vi "RT Loop - DAQ Control.vi"(11 "Message Queue":refnum<queue> caption="消息队列") -> ()   [LabVIEW 2013]
doc: "该DAQ控制循环VI对4路输入通道并行地进行控制计算，将结果输出至输出通道。"
uses:
  support/Message Queue/Message Cluster.ctl
  <vilib>/Platform/TimedLoop/XDataNode/timing_clust.ctl
  <vilib>/Platform/TimedLoop/XDataNode/nitl_modes.ctl
  <vilib>/Platform/TimedLoop/XDataNode/wakeup.ctl
  controls/Functional Global Operation.ctl
  controls/Control State.ctl
  Globals/Global - Configuration Options.vi
  <vilib>/Platform/TimedLoop/XDataNode/XDataNode.xnode
  <vilib>/Platform/TimedLoop/XDataNode/XDNodeRunTimeDep.lvlib
  support/Message Queue/Message Queue.lvlib
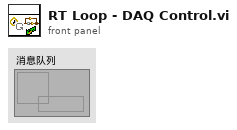
[diagram p1: front panel]
types:
  T1 = typedef "DAQ Tasks.ctl" = cluster{"AI Task":refnum<k21>, "AO Task":refnum<k21>}
  T2 = typedef "Functional Global Operation.ctl" = enum16{"Initialize", "Read", "Write"}
  T3 = typedef "XDNodeRunTimeDep.lvlib/timing_clust.ctl" = cluster{"Expected End [f-1]":u64, "Actual End [f-1]":u64, "Finished Late? [f-1]":bool, "Expected End [i-1]":u64, "Actual End [i-1]":u64, "Finished Late? [i-1]":bool, "Expected Start [i]":u64, "Actual Start [i]":u64, "Expected Start [f]":u64, "Actual Start [f]":u64, "Source Name":string, "Structure Name":string, "Period":i64, "Deadline":i64, "Offset":i64, "Start":i64, "Priority":i32, "Timeout":i32, "Mode":T4, "Wakeup Reason":T5, "Error":errorcluster, "Source Type":string, "Secondary Source Type":string, "Global End Time":u64, "Global Start Time":u64, "Frame Duration":u64, "Iteration Duration":u64, "Assigned CPU":i32, "I/O Scan Engine Mode":u32}
  T4 = typedef "XDNodeRunTimeDep.lvlib/nitl_modes.ctl" = enum32{"No Change", "Process missed periods, maintain original phase", "Discard missed periods, maintain original phase", "Process missed periods, ignore original phase", "Discard missed periods, ignore original phase"}
  T5 = typedef "XDNodeRunTimeDep.lvlib/wakeup.ctl" = enum32{"Normal", "Aborted", "Asynchronous wakeup", "Timing source error", "Timed loop error", "Timeout"}
  T6 = typedef "Control State.ctl" = enum16{"Safe State", "Manual", "Control (PID)"}
  T7 = typedef "Control Configuration.ctl" = cluster{"PID Gains":cluster{"proportional gain (Kc)":dbl, "integral gain (Kc*Ts/Ti)":dbl, "derivative gain (Kc*Td/Ts)":dbl}, "Output Range":cluster{"output high":dbl, "output low":dbl}}
  T8 = cluster{"proportional gain (Kc)":dbl, "integral gain (Kc*Ts/Ti)":dbl, "derivative gain (Kc*Td/Ts)":dbl}
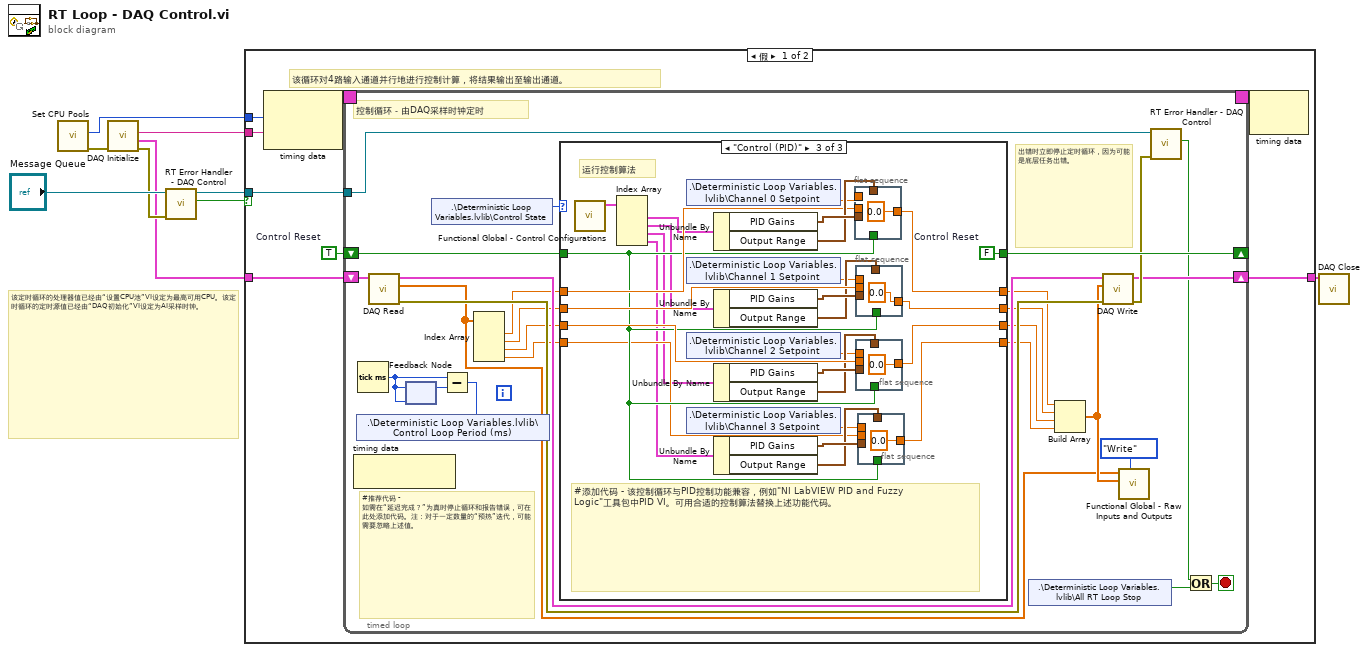
[diagram p0: block diagram]
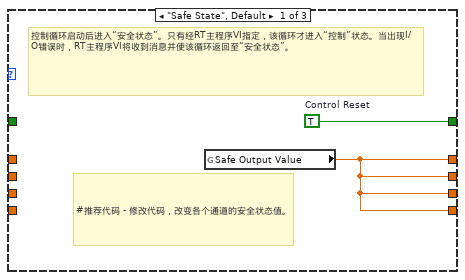
[diagram p2: hidden frame]
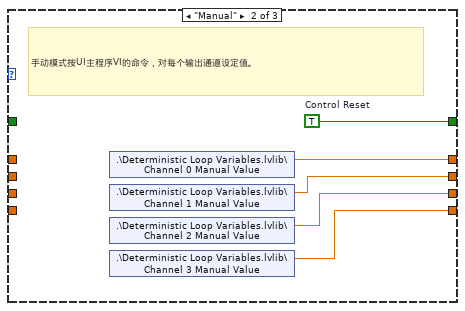
[diagram p3: hidden frame]
diagram:
  # "该定时循环的处理器值已经由“设置CPU池”VI设定为最高可用CPU。该定时循环的定时源值已经由“DAQ初始化”VI设定为AI采样时钟。"
  n1 = call "Set CPU Pools.vi"() -> ("error out"=w3:errorcluster, "Processor Assignment"=w2:i32)  [unwired: 10 in]
  n2 = call "DAQ Initialize.vi"("error in (no error)"=w3) -> ("error out"=w7:errorcluster, "DAQ Tasks"=w5:T1, "Timing Source"=w6:string)  [unwired: 8 in]
  n3 = call "RT Error Handler - DAQ Control.vi"("error in (no error)"=w7, "Message Queue"="Message Queue") -> ("Enqueued Error?"=w1:bool, "dup Message Queue"=w8:refnum<queue>)  [unwired: 8 in]
  n4 = case shown="假" w1 {
    tunnel: w8 -> [w14 _]
    tunnel: w6 -> [w13 _]
    tunnel: w5 -> [w12 w89]
    tunnel: [w11 w89] -> w4
    tunnel: w2 -> [w10 _]
    frame False {
      w15 = TRUE  # Control Reset
      # "该循环对4路输入通道并行地进行控制计算，将结果输出至输出通道。"
      n5 = node-c288(w10, w13) -> (w17:T3)
      n6 = timed-loop {
        shift-right: [w43] -> _
        shift-left: w15 -> [w42]
        timing: w17 -> [_]
        timing-out: [_] -> w16
        tunnel: w14 -> [w41]
        shift-right: [w31] -> w11
        shift-left: w12 -> [w33]
        stop <- w19 stop-if-true
        # "出错时立即停止定时循环，因为可能是底层任务出错。"
        # "#推荐代码 - 如需在“延迟完成？”为真时停止循环和报告错误，可在此处添加代码。注：对于一定数量的“预热”迭代，可能需要忽略上述值。"
        # "控制循环－由DAQ采样时钟定时"
        n7 = node-c288() -> ()  [unwired: 1 in, 1 out]
        n8 = Tick Count (ms)() -> (millisecond timer value=w40:u32)
        n9 = call "DAQ Read.vi"("DAQ Tasks"=w33) -> ("error out"=w34:errorcluster, "data"=w20:dbl[], "dup DAQ Tasks"=w32:T1)  [unwired: 8 in]
        n10 = feedback-in #1(w40) -> ()
        n11 = feedback #1(w40) -> (w39:u32)
        n12 = shared-variable ".\\Deterministic Loop Variables.lvlib\\Control State"() -> (w36:T6)  [unwired: 1 in, 1 out]
        n13 = Subtract(x=w40, y=w39) -> (x-y=w37:u32)
        n14 = shared-variable ".\\Deterministic Loop Variables.lvlib\\Control Loop Period (ms)"(w37) -> ()  [unwired: 1 in, 1 out]
        n15 = Index Array(array=w20) -> (element #1=w24:dbl, element #2=w23:dbl, element #3=w22:dbl, element #4=w21:dbl)  [unwired: 4 in]
        n16 = case shown="\"Control (PID)\"" w36 {
          tunnel: w24 -> [_ _ w74]
          tunnel: [w45 w50 w77] -> w28
          tunnel: [w46 w51 w78] -> w43
          tunnel: w42 -> [_ _ w62]
          tunnel: w23 -> [_ _ w73]
          tunnel: w22 -> [_ _ w69]
          tunnel: w21 -> [_ _ w61]
          tunnel: [w45 w49 w71] -> w27
          tunnel: [w45 w48 w66] -> w26
          tunnel: [w45 w47 w63] -> w25
          frame "Safe State", Default {
            w46 = TRUE  # Control Reset
            # "控制循环启动后进入“安全状态”。只有经RT主程序VI指定，该循环才进入“控制”状态。当出现I/O错误时，RT主程序VI将收到消息并使该循环返回至“安全状态”。"
            # "安全状态－下一个状态改变前，输出常量值"
            # "#推荐代码 - 修改代码，改变各个通道的安全状态值。"
            n17 = global read "Global - Configuration Options.vi" "Safe Output Value"() -> (w45:dbl)
          }
          frame "Manual" {
            w51 = TRUE  # Control Reset
            # "手动模式按UI主程序VI的命令，对每个输出通道设定值。"
            # "安全状态－下一个状态改变前，输出常量值"
            n18 = shared-variable ".\\Deterministic Loop Variables.lvlib\\Channel 0 Manual Value"() -> (w50:dbl)  [unwired: 1 in, 1 out]
            n19 = shared-variable ".\\Deterministic Loop Variables.lvlib\\Channel 1 Manual Value"() -> (w49:dbl)  [unwired: 1 in, 1 out]
            n20 = shared-variable ".\\Deterministic Loop Variables.lvlib\\Channel 2 Manual Value"() -> (w48:dbl)  [unwired: 1 in, 1 out]
            n21 = shared-variable ".\\Deterministic Loop Variables.lvlib\\Channel 3 Manual Value"() -> (w47:dbl)  [unwired: 1 in, 1 out]
          }
          frame "Control (PID)" {
            w78 = FALSE  # Control Reset
            # "运行控制算法"
            # "#添加代码 - 该控制循环与PID控制功能兼容，例如\"NI LabVIEW PID and Fuzzy Logic\"工具包中PID VI。可用合适的控制算法替换上述功能代码。"
            n22 = call "Functional Global - Control Configurations.vi"() -> ("Control Configurations out"=w60:T7[])  [unwired: 11 in]
            n23 = Index Array(array=w60) -> (element #1=w59:T7, element #2=w58:T7, element #3=w57:T7, element #4=w56:T7)  [unwired: 4 in]
            n24 = shared-variable ".\\Deterministic Loop Variables.lvlib\\Channel 0 Setpoint"() -> (w52:dbl)  [unwired: 1 in, 1 out]
            n25 = shared-variable ".\\Deterministic Loop Variables.lvlib\\Channel 1 Setpoint"() -> (w53:dbl)  [unwired: 1 in, 1 out]
            n26 = shared-variable ".\\Deterministic Loop Variables.lvlib\\Channel 2 Setpoint"() -> (w54:dbl)  [unwired: 1 in, 1 out]
            n27 = shared-variable ".\\Deterministic Loop Variables.lvlib\\Channel 3 Setpoint"() -> (w55:dbl)  [unwired: 1 in, 1 out]
            n28 = Unbundle By Name(w59) -> ("PID Gains"=w76:T8, "Output Range"=w75:cluster{"output high":dbl, "output low":dbl})
            n29 = Unbundle By Name(w58) -> ("PID Gains"=w72:T8, "Output Range"=w70:cluster{"output high":dbl, "output low":dbl})
            n30 = Unbundle By Name(w57) -> ("PID Gains"=w68:T8, "Output Range"=w67:cluster{"output high":dbl, "output low":dbl})
            n31 = Unbundle By Name(w56) -> ("PID Gains"=w65:T8, "Output Range"=w64:cluster{"output high":dbl, "output low":dbl})
            n32 = flat-sequence {
              tunnel: [0.0 ("output")] -> w77
              tunnel: w76 -> [_]
              tunnel: w75 -> [_]
              tunnel: w74 -> [_]
              tunnel: w62 -> [_]
              tunnel: w52 -> [_]
              frame #0 {
              }
            }
            n33 = flat-sequence {
              tunnel: w73 -> [_]
              tunnel: w72 -> [_]
              tunnel: [0.0 ("output")] -> w71
              tunnel: w70 -> [_]
              tunnel: w62 -> [_]
              tunnel: w53 -> [_]
              frame #0 {
              }
            }
            n34 = flat-sequence {
              tunnel: w69 -> [_]
              tunnel: w68 -> [_]
              tunnel: w67 -> [_]
              tunnel: [0.0 ("output")] -> w66
              tunnel: w62 -> [_]
              tunnel: w54 -> [_]
              frame #0 {
              }
            }
            n35 = flat-sequence {
              tunnel: w65 -> [_]
              tunnel: w64 -> [_]
              tunnel: [0.0 ("output")] -> w63
              tunnel: w62 -> [_]
              tunnel: w61 -> [_]
              tunnel: w55 -> [_]
              frame #0 {
              }
            }
          }
        }
        n36 = shared-variable ".\\Deterministic Loop Variables.lvlib\\All RT Loop Stop"() -> (w38:bool)  [unwired: 1 in, 1 out]
        n37 = Build Array(w28, w27, w26, w25) -> (w29:dbl[])
        n38 = call "DAQ Write.vi"("error in (no error)"=w34, "Outputs"=w29, "DAQ Tasks"=w32) -> ("error out"=w35:errorcluster, "dup DAQ Tasks"=w31:T1)  [unwired: 7 in]
        n39 = call "Functional Global - Raw Inputs and Outputs.vi"("Functional Global Operation (Read)"=Functional_Global_Operation."Write", "Outputs in"=w29, "Inputs in"=w20) -> ()  [unwired: 7 in, 2 out]
        n40 = call "RT Error Handler - DAQ Control.vi"("error in (no error)"=w35, "Message Queue"=w41) -> ("Enqueued Error?"=w18:bool)  [unwired: 8 in, 1 out]
        n41 = Or(x=w18, y=w38) -> (x .or. y?=w19:bool)
      }
      n42 = node-c288(w16) -> ()  [unwired: 1 out]
    }
    frame True {
      # "如设置DAQ任务时出错，不执行定时循环，直接关闭各任务。"
    }
  }
  n43 = call "DAQ Close.vi"("DAQ Tasks"=w4) -> ()  [unwired: 10 in, 1 out]
